vi "Cont Gen Voltage Wfm-Int Clk-Non Regeneration.vi"() -> ()   [LabVIEW 2021]
doc: "I. Description:\nThis example demonstrates how to continuously output a waveform using an internal sample clock. The automatic regeneration of data has been disabled, so new data has to be provided throughout the duration of the continuous Analog Output operation. This allows the generation of any arbitrary frequency as this VI computes new data for each iteration of the loop, maintaining phase continuity of the signal.\n\nII. Instructions for Running:\n1. Select the Physical Channel to correspond to where your signal is output on the DAQ device.\n2. Enter the Minimum and Maximum Voltage range.\n3. Specify the desired Sample Clock Rate of the output Waveform. Higher sample clock rates will produce a smoother waveform.\n4. Manually specify the Analog Output buffer size, in number of samples. A larger buffer would help non-regenerative operations avoid errors due to occasional high CPU load. \nNote: \nThe Analog Output buffer has to be at least as big as the amount of data being written to the board per iteration. The recommended buffer size would be at least twice the amount of data being written to the board per iteration.\n5. Enter the Waveform Information. See the documentation of the Basic Function Generator SubVI for information on each parameter.\n\nIII. Block Diagram Steps:\n1. Create an Analog Output Voltage channel.\n2. Configure the task to prohibit the automatic regeneration of data.\n3. Call the DAQmx (Sample Clock) VI to set the sample clock rate. Additionally, set the sample mode to Continuous.\n4. Read the actual sample clock rate (eventually coerced depending on the hardware used). \n5. Compute the desired waveform, using the buffer size and the actual update rate. This VI keeps track of the phase of the waveform to ensure that the generated signal is continuous.\n6. Write the waveform to the output buffer. \n7a. Call the Start VI. This is only needed when the loop is executed for the first time.\n7b. Do nothing.\n8. Loop continuously until user presses the Stop button. Every iteration computes and writes a new waveform to the buffer.\n9. Call the Clear Task VI to clear the Task.\n10. Use the popup dialog box to display an error or warning if any.\n\nIV. I/O Connections Overview:\nMake sure your signal output terminal matches the Physical Channel I/O Control. For further connection information, refer to your hardware reference manual."
uses:
  <vilib>/userdefined/High Color/nirio_resource_hc.ctl
  <vilib>/FPGAPlugInAG/PCIe-7857/niLvFpga_Open_PCIe-7857.vi
  <vilib>/rvi/interface/common/dynamic/niFpgaDynamicAddResources.vi
  <vilib>/Utility/error.llb/Error Cluster From Error Code.vi
  <vilib>/rvi/errors/niLvFpgaAdjustHostInterfaceError.vi
  <vilib>/rvi/interface/common/niFpgaWaitOnOcc.vi
  <vilib>/FPGAPlugInAG/Dynamic/niLvFpga_Run_Dynamic.vi
  <vilib>/FPGAPlugInAG/Dynamic/niLvFpga_Close_Dynamic.vi
  <vilib>/rvi/interface/nirviOpenFPGA/nirviOpenFPGA.xnode
  FPGA Bitfiles/lvfpga_FPGATarget_AO_PspK-PiI6Y0.lvbitx
  output_FPGA.vi
  <vilib>/rvi/interface/nirviReadWriteControl/nirviReadWriteControl.xnode
  <vilib>/rvi/interface/nirviMethod/nirviMethod.xnode
  <vilib>/rvi/interface/nirviCloseFPGA/nirviCloseFPGA.xnode
  <vilib>/measure/NI_MABase.lvlib
  <vilib>/rvi/errors/niLvFpgaMergeErrorWithErrorCode.vi
  <vilib>/rvi/interface/Simulation/niFpgaSimulationCallBeginRW.vi
  <vilib>/FPGAPlugInAG/Dynamic/niLvFpga_WriteFifo_Dynamic.vi
  NiFpgaLv.dll
  <vilib>/FPGAPlugInAG/Dynamic/niLvFpga_ConfigureFifo_Dynamic.vi
panel:
  in  "RIO Resource Name":T1="RIO0" caption="RIO Device"
  in  "Size (Samples)":u32=5000
  out "Actual Sample Clock Rate":dbl=20000.0 format="%.2f"
  in  "Sample Clock Rate":dbl=200.0 format="%0.2f"
  in  "Waveform Type":T2(ring)
  in  "Frequency":dbl=997.0 format="%.2f"
  in  "Amplitude":dbl=1.0 format="%0.2p"
  in  "stop":bool
  # "Channel Parameters"
  # "RIO0::INSTR"
  # "Timing Parameters"
  # "Waveform Information"
  # "Buffer Parameters"
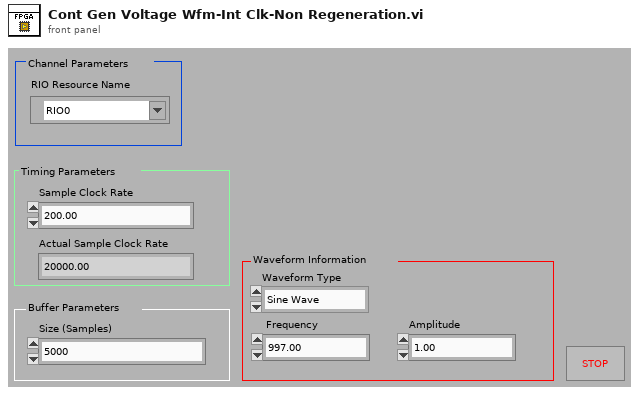
[diagram p1: front panel]
types:
  T1 = typedef "nirio_resource_hc.ctl" = tag
  T2 = enum16{"Sine Wave", "Triangle Wave", "Square Wave", "Sawtooth Wave"}
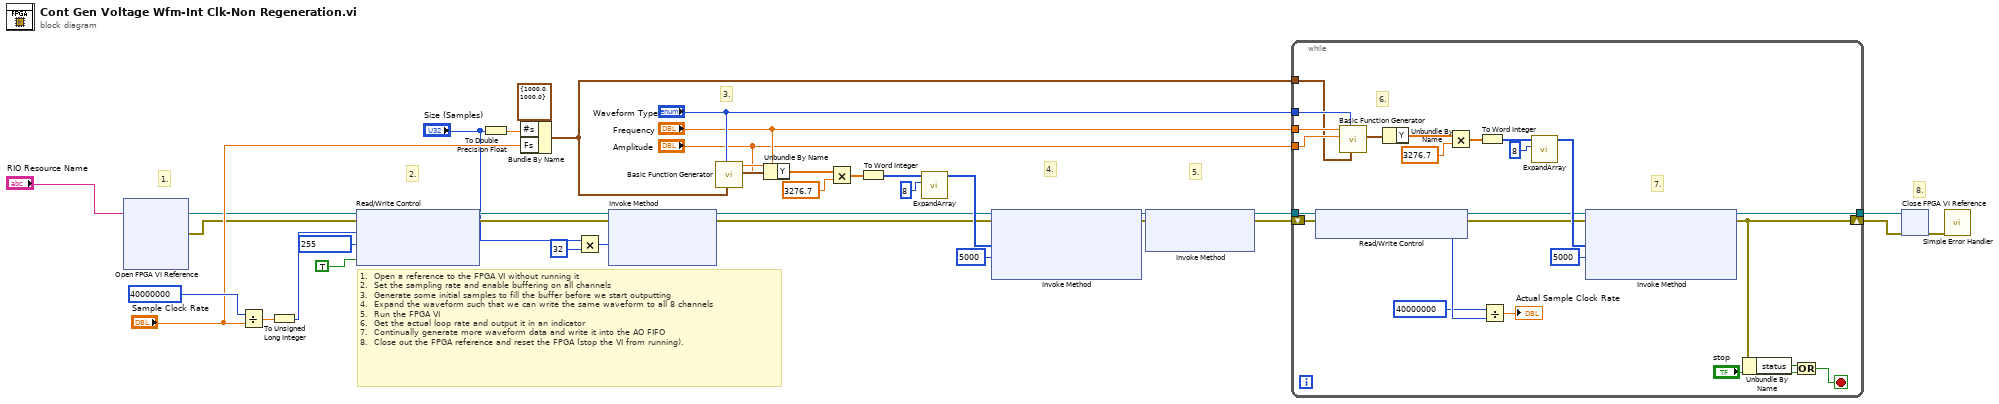
[diagram p0: block diagram]
diagram:
  # "1.  Open a reference to the FPGA VI without running it\n2.  Set the sampling rate and enable buffering on all channels\n3.  Generate some initial samples to fill the buffer before we start outputting\n4.  Expand the waveform such that we can write the same waveform to all 8 channels\n5.  Run the FPGA VI\n6.  Get the actual loop rate and output it in an indicator\n7.  Continually generate more waveform data and write it into the AO FIFO\n8.  Close out the FPGA reference and reset the FPGA (stop the VI from running)."
  # "8."
  # "5."
  # "4."
  # "3."
  # "2."
  # "1."
  n1 = xnode "Open FPGA VI Reference"("resource name"="RIO Resource Name") -> ("FPGA VI Reference Out"=w2:refnum<k20>, "error out"=w1:errorcluster)  [unwired: 1 in]
  n2 = Divide(x=u32 40000000, y="Sample Clock Rate") -> (x/y=w35:dbl)
  n3 = To Unsigned Long Integer(number=w35) -> (unsigned 32bit integer=w34:u32)
  n4 = xnode "Read/Write Control"("FPGA VI Reference In"=w2, "error in"=w1, "AO Loop Timer(Ticks)"=w34, "AO Buffer Enable"=u8 255, "AO Enable"=TRUE) -> ("FPGA VI Reference Out"=w10:refnum<k20>, "error out"=w9:errorcluster)
  n5 = To Double Precision Float(number="Size (Samples)") -> (double precision float=w30:dbl)
  n6 = Bundle By Name(cluster=cluster{"Fs":dbl, "#s":dbl} {"Fs"=1000.0, "#s"=1000.0} ("sampling info"), "#s"=w30, "Fs"="Sample Clock Rate") -> (w21:cluster{"Fs":dbl, "#s":dbl})
  n7 = Multiply(x="Size (Samples)", y=u32 32) -> (x*y=w4:u32)
  n8 = xnode "Invoke Method"("FPGA VI Reference In"=w10, "error in"=w9, "Requested Depth"=w4) -> ("FPGA VI Reference Out"=w8:refnum<k20>, "error out"=w7:errorcluster)  [unwired: 1 out]
  n9 = call <vilib>:"Basic Function Generator.vi"("sampling info"=w21, "signal type"="Waveform Type", "amplitude"="Amplitude", "frequency"="Frequency") -> ("signal out"=w29:waveform(dbl))  [unwired: 5 in, 2 out]
  n10 = Unbundle By Name(w29) -> ("Y"=w28:dbl[])
  n11 = Multiply(x=w28, y=3276.7) -> (x*y=w26:dbl[])
  n12 = To Word Integer(number=w26) -> (16bit integer=w17:i16[])
  n13 = call "ExpandArray.vi"("Scale Factor"=u16 8, "Input AO Array"=w17) -> ("Output Array"=w16:i16[])  [unwired: 9 in]
  n14 = xnode "Invoke Method"("FPGA VI Reference In"=w8, "error in"=w7, "Data"=w16, "Timeout (ms)"=5000) -> ("FPGA VI Reference Out"=w24:refnum<k20>, "error out"=w11:errorcluster)  [unwired: 1 out]
  n15 = xnode "Invoke Method"("FPGA VI Reference In"=w24, "error in"=w11) -> ("FPGA VI Reference Out"=w23:refnum<k20>, "error out"=w22:errorcluster)  [unwired: 1 in]
  n16 = while {
    tunnel: w23 -> [w48]
    shift-right: [w39] -> w13
    shift-left: w22 -> [w47]
    tunnel: w21 -> [w58]
    tunnel: "Waveform Type" -> [w61]
    tunnel: "Frequency" -> [w60]
    tunnel: "Amplitude" -> [w59]
    tunnel: [w50] -> w14
    stop <- w40 stop-if-true
    # "7."
    # "6."
    n17 = xnode "Read/Write Control"("FPGA VI Reference In"=w48, "error in"=w47) -> ("FPGA VI Reference Out"=w46:refnum<k20>, "error out"=w45:errorcluster, "AO: Actual Loop Rate(ticks)"=w44:u32)
    n18 = call <vilib>:"Basic Function Generator.vi"("sampling info"=w58, "signal type"=w61, "amplitude"=w59, "frequency"=w60) -> ("signal out"=w54:waveform(dbl))  [unwired: 5 in, 2 out]
    n19 = Unbundle By Name(w54) -> ("Y"=w57:dbl[])
    n20 = Multiply(x=w57, y=3276.7) -> (x*y=w55:dbl[])
    n21 = To Word Integer(number=w55) -> (16bit integer=w53:i16[])
    n22 = Divide(x=u32 40000000, y=w44) -> (x/y=→"Actual Sample Clock Rate":dbl)
    n23 = call "ExpandArray.vi"("Scale Factor"=u16 8, "Input AO Array"=w53) -> ("Output Array"=w51:i16[])  [unwired: 9 in]
    n24 = xnode "Invoke Method"("FPGA VI Reference In"=w46, "error in"=w45, "Data"=w51, "Timeout (ms)"=5000) -> ("FPGA VI Reference Out"=w50:refnum<k20>, "error out"=w39:errorcluster)  [unwired: 1 out]
    n25 = Unbundle By Name(w39) -> ("status"=w38:bool)
    n26 = Or(x=w38, y="stop") -> (x .or. y?=w40:bool)
  }
  n27 = xnode "Close FPGA VI Reference"("FPGA VI Reference In"=w14, "error in"=w13) -> ("error out"=w12:errorcluster)
  n28 = call <vilib>:"Simple Error Handler.vi"("error in (no error)"=w12) -> ()  [unwired: 4 in, 5 out]
